vi "GetAttributeViInt32_SA-HD_OB.vi"(8 "error in (no error)":errorcluster {"code" format="%.0x"}, 9 "AttributeID":u32(ring)=1150456 items=["SA_HARMONICDISTORTION_AVERAGE_COUNT"=1150456, "SA_HARMONICDISTORTION_AVERAGE_MODE"=1150458, "SA_HARMONICDISTORTION_DISPLAYWINDOWY_REF_POSITION"=1150478, "SA_HARMONICDISTORTION_FREQUENCY_STEP"=1150462, "SA_HARMONICDISTORTION_NUMBER_OF_HARMONICS"=1150459, "SA_HARMONICDISTORTION_TRACE_TYPE"=1150777, "SA_HARMONICDISTORTION_TRIGGER_SOURCE"=1150470, "SA_OCCUPIEDBANDWIDTH_AVERAGE_COUNT"=1150289, "SA_OCCUPIEDBANDWIDTH_AVERAGE_MODE"=1150291, "SA_OCCUPIEDBANDWIDTH_DETECTOR_TYPE"=1150286, "SA_OCCUPIEDBANDWIDTH_DISPLAY_BOUNDARY_FREQUENCY_DISPLAY_TYPE"=1150871, "SA_OCCUPIEDBANDWIDTH_DISPLAY_VIEW_SELECTION"=1150869, "SA_OCCUPIEDBANDWIDTH_DISPLAY_WINDOWY_REF_POSITION"=1150310, "SA_OCCUPIEDBANDWIDTH_MARKER_ACTIVE_MARKER"=1150321, "SA_OCCUPIEDBANDWIDTH_MARKER_COUNT"=1150323, "SA_OCCUPIEDBANDWIDTH_MARKER_DELTA_REFERENCE"=1150325, "SA_OCCUPIEDBANDWIDTH_MARKER_TYPE"=1150330, "SA_OCCUPIEDBANDWIDTH_POWER_REFERENCE_TYPE"=1150827, "SA_OCCUPIEDBANDWIDTH_SWEEPCOUPLING_BANDWIDTH_SHAPE"=1150293, "SA_OCCUPIEDBANDWIDTH_SWEEPCOUPLING_SWEEP_POINTS"=1150109, "SA_OCCUPIEDBANDWIDTH_SWEEPCOUPLING_SWEEP_TIME_AUTO_RULES"=1150314, "SA_OCCUPIEDBANDWIDTH_TRACES_TYPE"=1150779, "SA_OCCUPIEDBANDWIDTH_TRIGGER_SOURCE"=1150333], 11 "instrument handle":refnum<k15>) -> (0 "error out":errorcluster {"code" format="%.0x"}, 2 "AttributeValue":i32, 3 "instrument handle out":refnum<k15>)   [LabVIEW 2009, in "Keysight XSAn.lvlib"]
doc: "Gets an Int32 attribute from the instrument driver.\nThe following Attributes are supported:\n\nSA_HARMONICDISTORTION_AVERAGE_COUNT\nSA_HARMONICDISTORTION_AVERAGE_MODE\nSA_HARMONICDISTORTION_DISPLAYWINDOWY_REF_POSITION\nSA_HARMONICDISTORTION_FREQUENCY_STEP\nSA_HARMONICDISTORTION_NUMBER_OF_HARMONICS\nSA_HARMONICDISTORTION_TRACE_TYPE\nSA_HARMONICDISTORTION_TRIGGER_SOURCE\nSA_OCCUPIEDBANDWIDTH_AVERAGE_COUNT\nSA_OCCUPIEDBANDWIDTH_AVERAGE_MODE\nSA_OCCUPIEDBANDWIDTH_DETECTOR_TYPE\nSA_OCCUPIEDBANDWIDTH_DISPLAY_BOUNDARY_FREQUENCY_DISPLAY_TYPE\nSA_OCCUPIEDBANDWIDTH_DISPLAY_VIEW_SELECTION\nSA_OCCUPIEDBANDWIDTH_DISPLAY_WINDOWY_REF_POSITION\nSA_OCCUPIEDBANDWIDTH_MARKER_ACTIVE_MARKER\nSA_OCCUPIEDBANDWIDTH_MARKER_COUNT\nSA_OCCUPIEDBANDWIDTH_MARKER_DELTA_REFERENCE\nSA_OCCUPIEDBANDWIDTH_MARKER_TYPE\nSA_OCCUPIEDBANDWIDTH_POWER_REFERENCE_TYPE\nSA_OCCUPIEDBANDWIDTH_SWEEPCOUPLING_BANDWIDTH_SHAPE\nSA_OCCUPIEDBANDWIDTH_SWEEPCOUPLING_SWEEP_POINTS\nSA_OCCUPIEDBANDWIDTH_SWEEPCOUPLING_SWEEP_TIME_AUTO_RULES\nSA_OCCUPIEDBANDWIDTH_TRACES_TYPE\nSA_OCCUPIEDBANDWIDTH_TRIGGER_SOURCE"
uses:
  <instrlib>/Keysight XSAn/Keysight XSAn.lvlib
  AgXSAn.dll
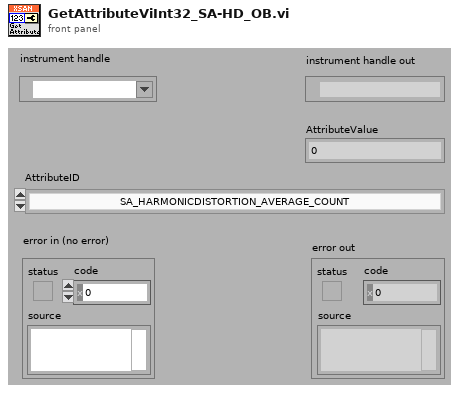
[diagram p1: front panel]
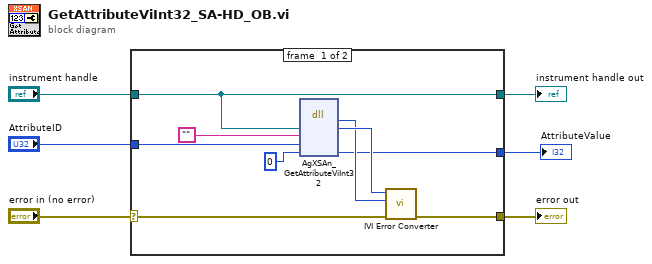
[diagram p0: block diagram]
diagram:
  n1 = case shown="No Error" "error in (no error)" {
    selector: "error in (no error)" -> [w13 w17]
    tunnel: [w12 w17] -> w6
    tunnel: "instrument handle" -> [w8 w16]
    tunnel: "AttributeID" -> [w11 _]
    tunnel: [w9 _] -> w2
    tunnel: [w8 w16] -> w1
    frame #0 {
      n2 = dll-call lib="AgXSAn**.dll" fn="AgXSAn_GetAttributeViInt32"("Vi"=w8, "RepCapIdentifier"="", "AttributeID"=w11, "AttributeValue"=0) -> ("return type"=w14:i32, "Vi"=w15:u32, "AttributeValue"=w9:i32)  [unwired: 5 in, 2 out]
      n3 = call <instrlib>:"IVI Error Converter.vi"("error in (no error)"=w13, "IVI error code (0)"=w14, "instrument handle"=w15) -> ("error out"=w12:errorcluster)  [unwired: 7 in, 1 out]
    }
    frame #1 {
    }
  }
  "error out" <- w6
  "instrument handle out" <- w1
  "AttributeValue" <- w2
